vi "SDCP SMF Receiver and Trasmitter - Live Plot - Backup - v2.vi"() -> ()   [LabVIEW 2020]
uses:
  Typedefs/SDCP - Standard Message Frame Parameters - FGV - commands.ctl
  Typedefs/SDCP - Serial Port Control - Commands.ctl
panel:
  in  "Zero offset":bool
  out "Adjusted Offset":dbl
  in  "Offset":dbl(c297)
  out "Active Plot Names":string[](array[string])
  out "Value":dbl
  out "Time (ms)":dbl
  in  "Cursor Parameter":string(combo)
  out "Instantaeneous data":T1(array[cluster])
  in  "Time span (ms)":dbl
  in  "Channel 8 enable":bool
  in  "Channel 7 enable":bool
  in  "Channel 6 enable":bool
  in  "Channel 5 enable":bool
  in  "Channel 4 enable":bool
  in  "Channel 3 enable":bool
  in  "Channel 2 enable":bool
  in  "Channel 1 enable":bool
  in  "Channel 8 parameter":string(combo)
  in  "Channel 7 parameter":string(combo)
  in  "Channel 6 parameter":string(combo)
  in  "Channel 5 parameter":string(combo)
  in  "Channel 4 parameter":string(combo)
  in  "Channel 3 parameter":string(combo)
  in  "Channel 2 parameter":string(combo)
  in  "Channel 1 parameter":string(combo)
  in  "Plot file path":path
  out "Live Plot":T2(graph)
  out "Time (ms)":u32
  in  "Stop Application":bool
  in  "Trace file path":path
  in  "Baud rate":u32=9600
  in  "COM Port":refnum<visa-resource-name>
  in  "Parameter file path":path=path "E:/Projects/System Diagnostics and Control Protocol/SDCP_LabVIEW/Parameter Files/Motion_Processing.param"
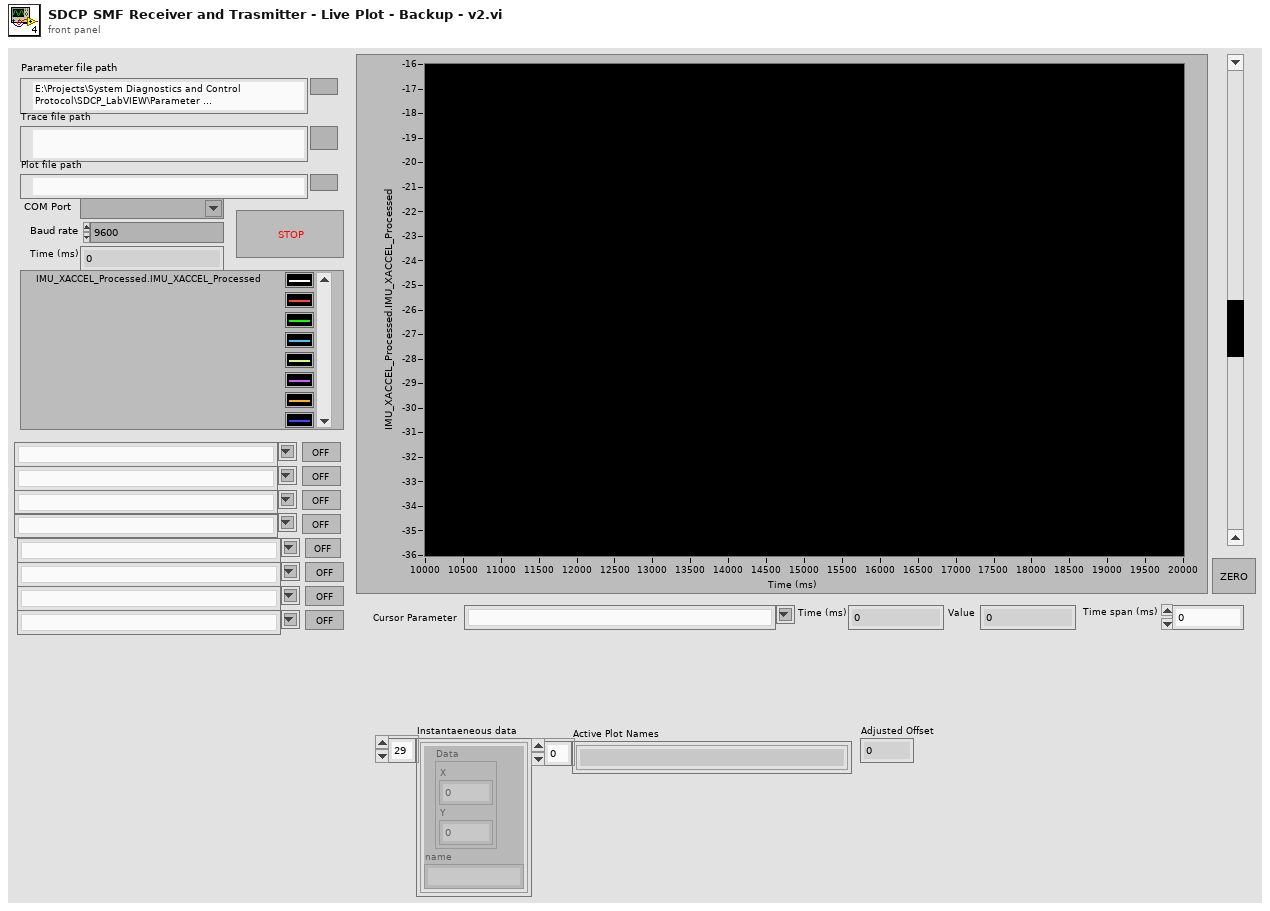
[diagram p1: front panel]
types:
  T1 = cluster{"Data":cluster{"X":dbl, "Y":dbl}, "name":string}[]
  T2 = cluster{"Plot data":cluster{"X":dbl, "Y":dbl}[]}[]
  T3 = typedef "SDCP - Serial Port Control - Commands.ctl" = enum16{"Open", "Read", "Write", "Get instance", "Close"}
  T4 = cluster{"data bytes":u8[], "Time (ms)":u32, "Direction":string}
  T5 = typedef "SDCP - Standard Message Frame Parameters - FGV - commands.ctl" = enum16{"Write descriptors", "Read descriptors", "Read values", "Load parameters from file", "Write values", "Read all descriptors"}
  T6 = typedef "SDCP - SMF parameter descriptors.ctl" = cluster{"Frame name":string, "Frame ID":i32, "Data type":string, "Start Position":i32, "Length":i32, "Factor":dbl, "Offset":dbl, "Parameter name":string, "Value":string}
  T7 = cluster{"name":string, "Data":cluster{"X":dbl, "Y":dbl}[]}
  T8 = cluster{"name":string, "Data":cluster{"X":dbl, "Y":dbl}[]}[]
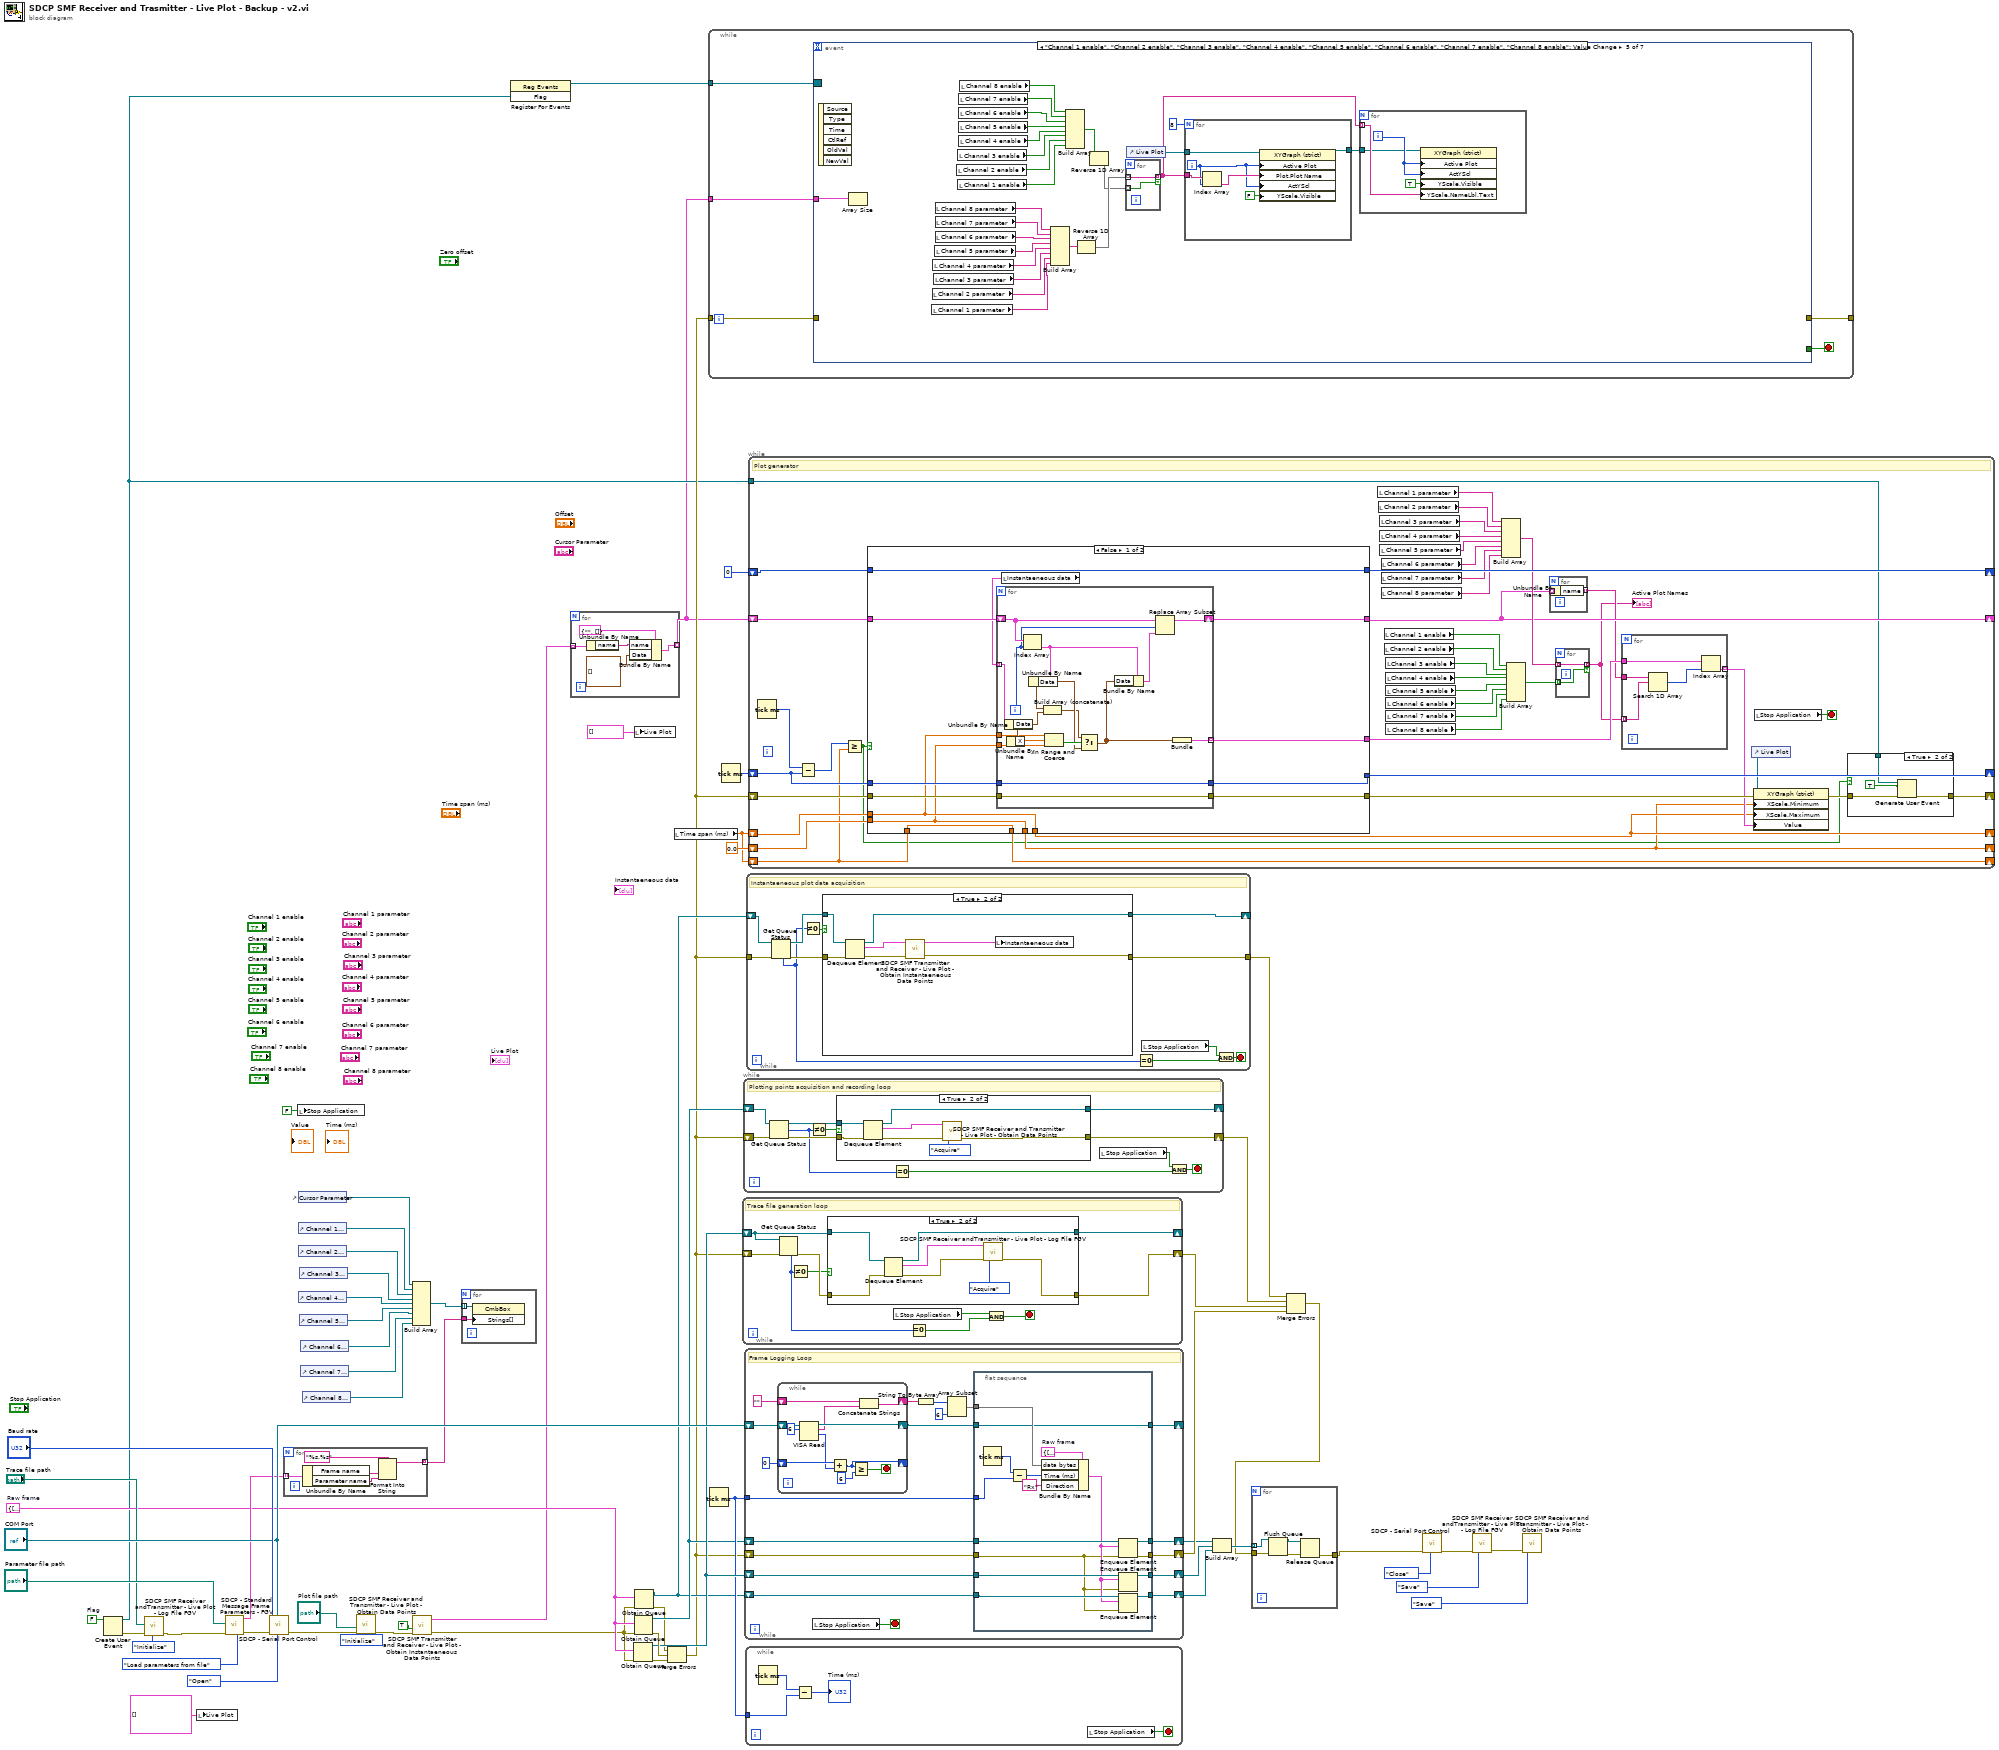
[diagram p0: block diagram]
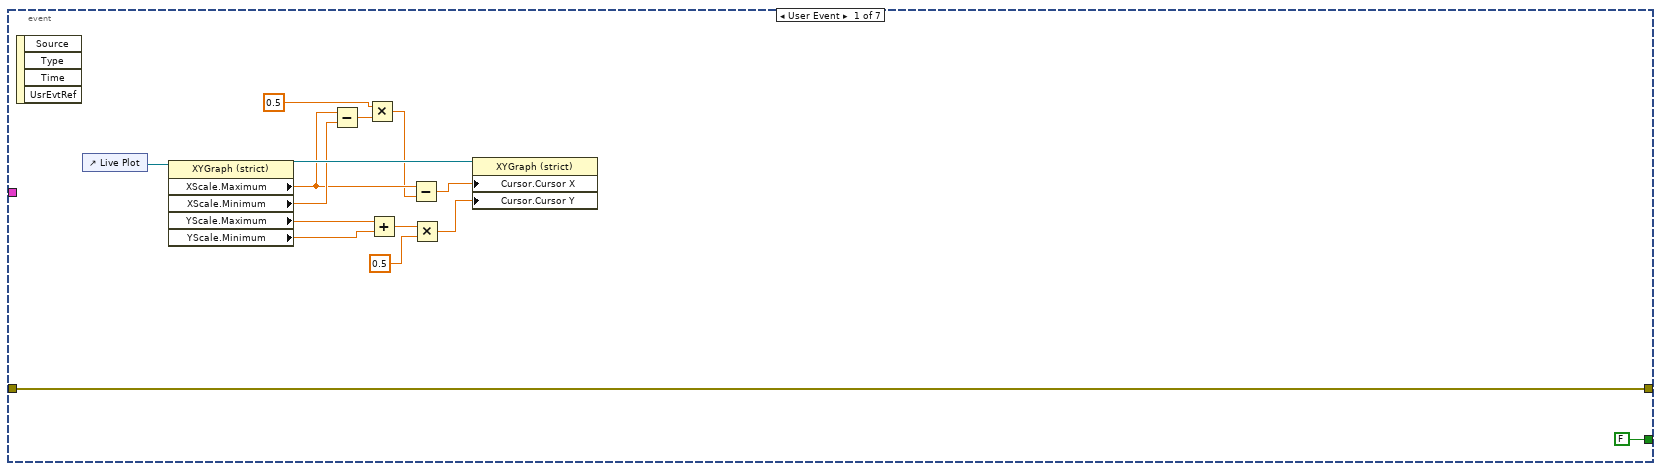
[diagram p2: hidden frame]
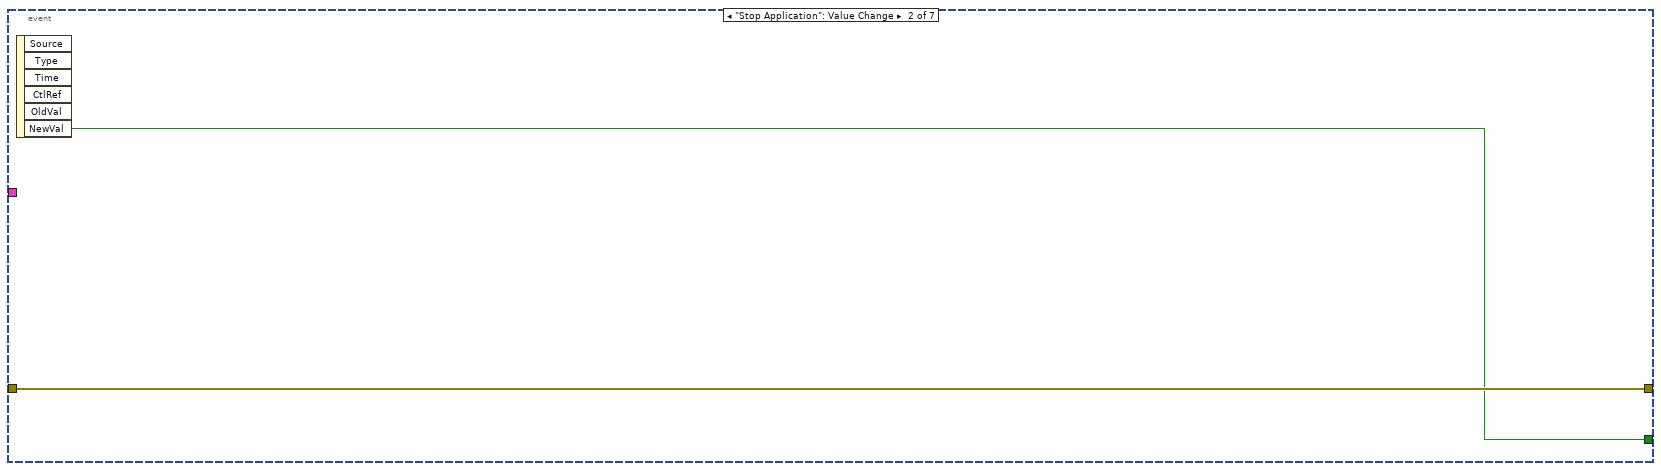
[diagram p3: hidden frame]
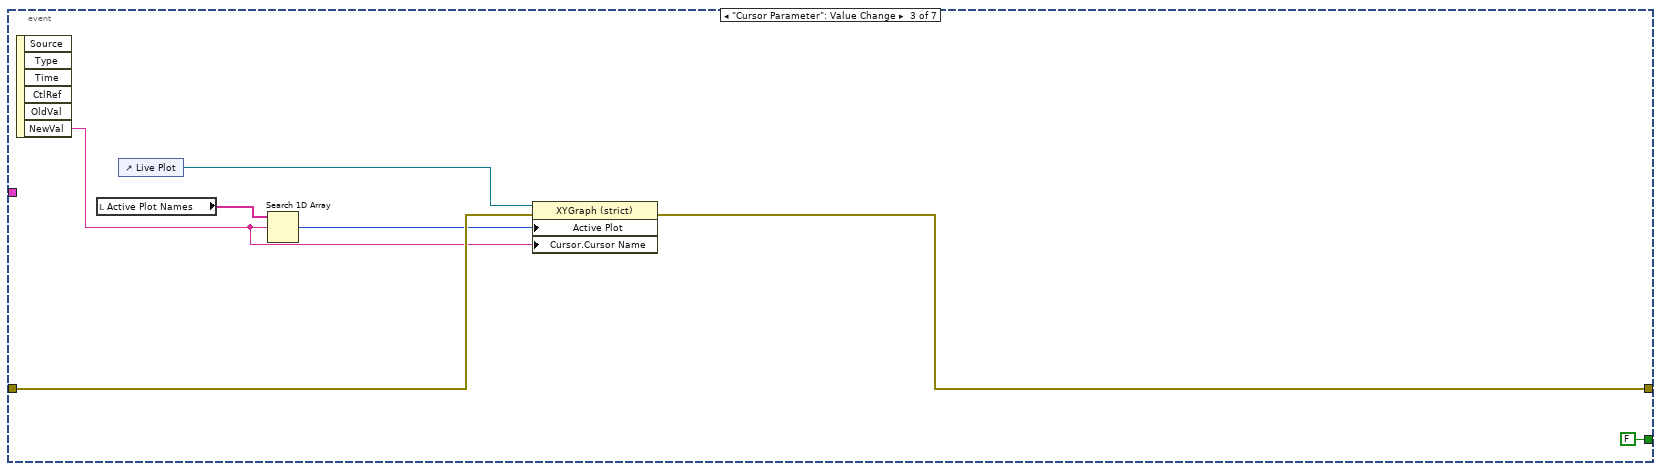
[diagram p4: hidden frame]
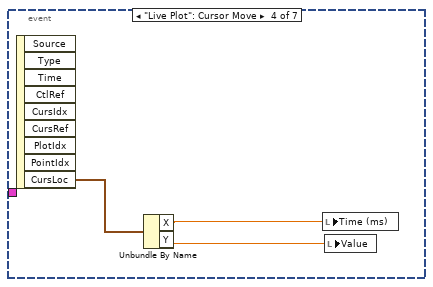
[diagram p5: hidden frame]
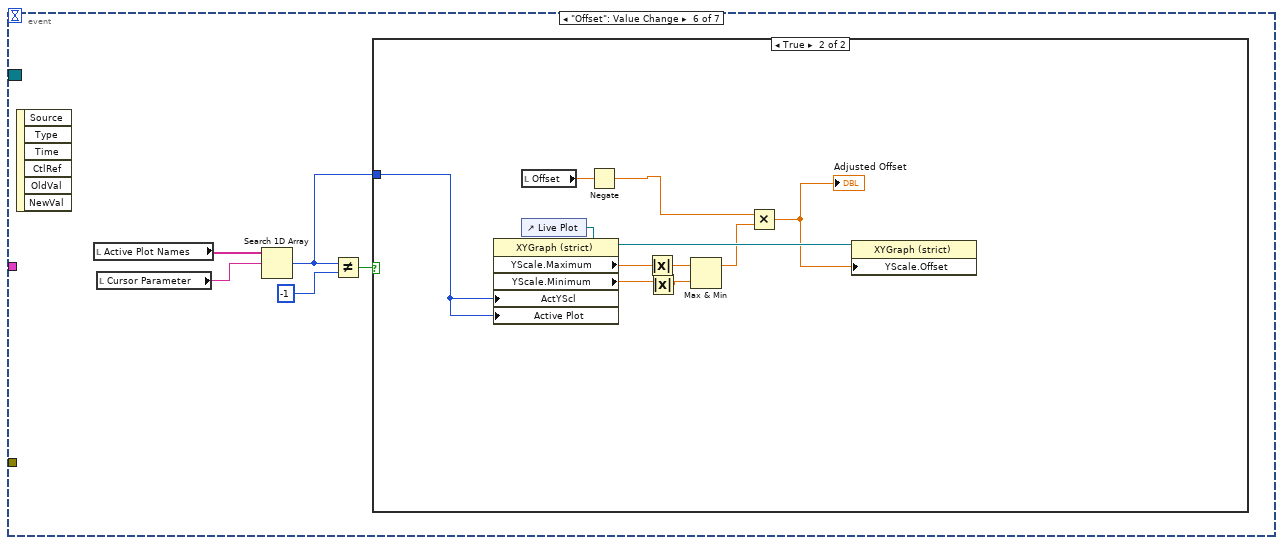
[diagram p6: hidden frame]
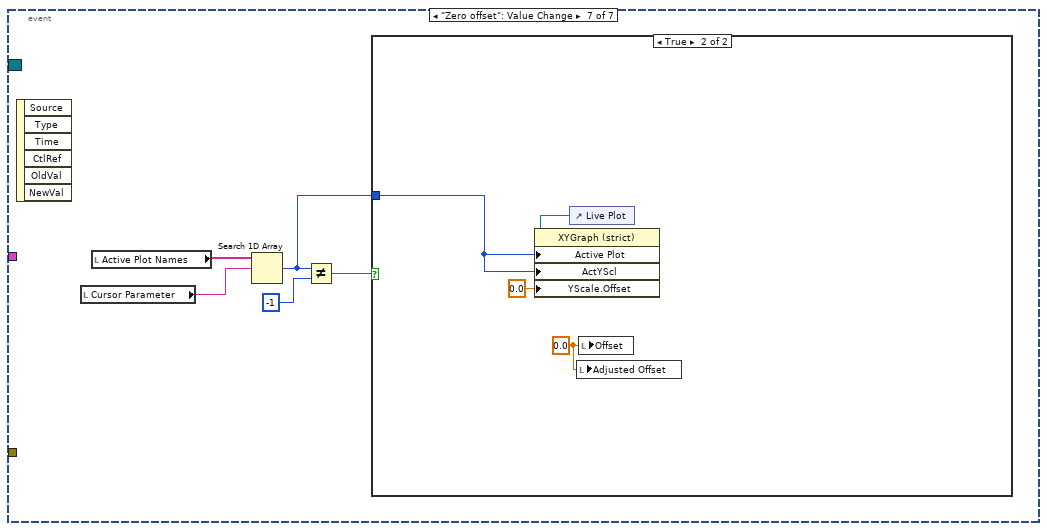
[diagram p8: hidden frame]
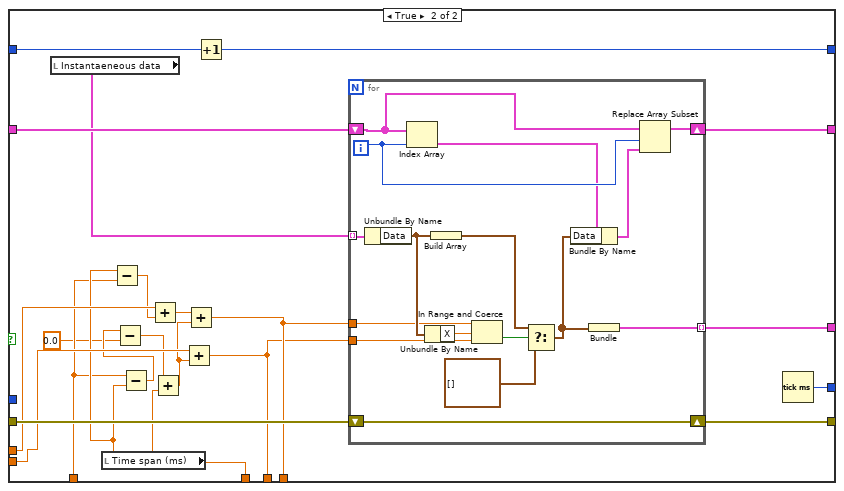
[diagram p11: hidden frame]
diagram:
  w4 = FALSE  # Flag
  w28 = T4 {"data bytes"=[], "Time (ms)"=0, "Direction"=""}  # Raw frame
  n1 = Create User Event(user event datatype=w4) -> (user event=w2:refnum<user-event>, error out=w5:errorcluster)  [unwired: 1 in]
  n2 = call "SDCP SMF Receiver andTransmitter - Live Plot - Log File FGV.vi"("error in (no error)"=w5, "Command"=enum16{"Initialize", "Acquire", "Save"}."Initialize", "Trace file path"="Trace file path") -> ("error out"=w46:errorcluster)  [unwired: 4 in]
  n3 = local write "Live Plot"(T2 [] ("Live Plot")) -> ()
  n4 = call "SDCP - Standard Message Frame Parameters - FGV.vi"("Parameter file path"="Parameter file path", "error in (no error)"=w46, "Command"=SDCP_-_Standard_Message_Frame_Parameters_-_FGV_-_commands."Load parameters from file") -> ("SMF Parameters descriptors out"=w41:T6[], "error out"=w62:errorcluster)  [unwired: 4 in]
  n5 = call "SDCP - Serial Port Control.vi"("Command"=SDCP_-_Serial_Port_Control_-_Commands."Open", "VISA resource name"="COM Port", "error in (no error)"=w62, "Baud rate"="Baud rate") -> ("error out"=w30:errorcluster)  [unwired: 4 in, 3 out]
  n6 = for {
    tunnel: w41 -> [w69] mode=indexing
    tunnel: [w65] -> w31 mode=indexing
    n7 = Unbundle By Name(w69) -> ("Frame name"=w67:string, "Parameter name"=w66:string)
    n8 = Format Into String(format string="%s.%s", w67, w66) -> (resulting string=w65:string)  [unwired: 2 in, 1 out]
  }
  n9 = local write "Stop Application"(FALSE ("Stop Application")) -> ()
  n10 = control-ref of="Cursor Parameter"() -> (w7:refnum<vi>)
  n11 = control-ref of="Channel 1 parameter"() -> (w40:refnum<vi>)
  n12 = control-ref of="Channel 2 parameter"() -> (w39:refnum<vi>)
  n13 = control-ref of="Channel 4 parameter"() -> (w37:refnum<vi>)
  n14 = control-ref of="Channel 3 parameter"() -> (w38:refnum<vi>)
  n15 = control-ref of="Channel 5 parameter"() -> (w36:refnum<vi>)
  n16 = control-ref of="Channel 6 parameter"() -> (w35:refnum<vi>)
  n17 = control-ref of="Channel 7 parameter"() -> (w34:refnum<vi>)
  n18 = control-ref of="Channel 8 parameter"() -> (w33:refnum<vi>)
  n19 = call "SDCP SMF Receiver and Transmitter - Live Plot - Obtain Data Points.vi"("error in (no error)"=w30, "Plot file path"="Plot file path", "Command"=enum16{"Initialize", "Acquire", "Save"}."Initialize") -> ("error out"=w17:errorcluster)  [unwired: 4 in]
  n20 = Build Array(w7, w40, w39, w38, w37, w36, w35, w34, w33) -> (w32:refnum<vi>[])
  n21 = call "SDCP SMF Transmitter and Receiver - Live Plot - Obtain Instantaeneous Data Points.vi"("Initialize ?"=TRUE, "error in (no error)"=w17) -> ("Instantaeneous data"=w13:T1, "error out"=w16:errorcluster)  [unwired: 4 in]
  n22 = for {
    tunnel: w32 -> [w71] mode=indexing
    tunnel: w31 -> [w70]
    n23 = property class="CmbBox"(reference=w71, "Strings[]"=w70) -> ()  [unwired: 1 in, 2 out]
  }
  n24 = register-events(w2) -> (reference out=w3:refnum<event-registration>)  [unwired: 2 in, 1 out]
  n25 = for {
    tunnel: w13 -> [w76] mode=indexing
    tunnel: [w73] -> w1 mode=indexing
    n26 = Unbundle By Name(w76) -> ("name"=w74:string)
    n27 = Bundle By Name(cluster=T7 {"name"="", "Data"=[]}, "name"=w74, "Data"=cluster{"X":dbl, "Y":dbl}[] []) -> (w73:T7)
  }
  n28 = Obtain Queue(element data type=w28, error in (no error)=w16) -> (queue out=w56:refnum<queue>, error out=w57:errorcluster)  [unwired: 3 in, 1 out]
  n29 = local write "Live Plot"(cluster{"Data":cluster{"X":dbl, "Y":dbl}[]}[] []) -> ()
  n30 = Obtain Queue(element data type=w28, error in (no error)=w16) -> (queue out=w47:refnum<queue>, error out=w58:errorcluster)  [unwired: 3 in, 1 out]
  n31 = Obtain Queue(element data type=w28, error in (no error)=w16) -> (queue out=w19:refnum<queue>, error out=w27:errorcluster)  [unwired: 3 in, 1 out]
  n32 = Merge Errors(w27, w58, w57) -> (w6:errorcluster)
  n33 = local read "Time span (ms)"() -> (w8:dbl)
  n34 = while {
    tunnel: w6 -> [w81]
    tunnel: [w80] -> _
    tunnel: w3 -> [w78]
    tunnel: w1 -> [w77]
    stop <- w79 stop-if-true
    n35 = event shown="[4] \"Channel 1 enable\", \"Channel 2 enable\", \"Channel 3 enable\", \"Channel 4 enable\", \"Channel 5 enable\", \"Channel 6 enable\", \"Channel 7 enable\", \"Channel 8 enable\": Value Change" {
      selector: w78 -> [_ _ _ _ _ _ _]
      dyn-events: _ -> [_ _ _ _ _ _ _]
      timeout: _ -> [_ _ _ _ _ _ _]
      tunnel: w81 -> [w96 w98 w104 _ _ _ _]
      tunnel: [w96 w98 w100 _ _ _ _] -> w80
      tunnel: [FALSE w97 FALSE ("NewVal") _ _ _ _] -> w79
      tunnel: w77 -> [_ _ _ _ w117 _ _]
      event User Event {
        n36 = event-data() -> ()  [unwired: 1 in, 4 out]
        n37 = control-ref of="Live Plot"() -> (w94:refnum<vi>)
        n38 = property class="XYGraph (strict)"(reference=w94) -> (reference out=w89:refnum<vi>, "XScale.Maximum"=w86:dbl, "XScale.Minimum"=w87:dbl, "YScale.Maximum"=w93:dbl, "YScale.Minimum"=w92:dbl)  [unwired: 1 in, 1 out]
        n39 = Subtract(x=w86, y=w87) -> (x-y=w85:dbl)
        n40 = Multiply(x=0.5, y=w85) -> (x*y=w83:dbl)
        n41 = Add(x=w93, y=w92) -> (x+y=w91:dbl)
        n42 = Subtract(x=w86, y=w83) -> (x-y=w82:dbl)
        n43 = Multiply(x=w91, y=0.5) -> (x*y=w88:dbl)
        n44 = property class="XYGraph (strict)"(reference=w89, "Cursor.Cursor X"=w82, "Cursor.Cursor Y"=w88) -> ()  [unwired: 1 in, 2 out]
      }
      event "Stop Application": Value Change {
        n45 = event-data() -> ("NewVal"=w97:bool)  [unwired: 1 in, 5 out]
      }
      event "Cursor Parameter": Value Change {
        n46 = event-data() -> ("NewVal"=w101:string)  [unwired: 1 in, 5 out]
        n47 = local read "Active Plot Names"() -> (w99:string[])
        n48 = control-ref of="Live Plot"() -> (w103:refnum<vi>)
        n49 = Search 1D Array(1D array=w99, element=w101) -> (index of element=w102:i32)  [unwired: 1 in]
        n50 = property class="XYGraph (strict)"(reference=w103, error in=w104, "Active Plot"=w102, "Cursor.Cursor Name"=w101) -> (error out=w100:errorcluster)  [unwired: 1 out]
      }
      event "Live Plot": Cursor Move {
        n51 = event-data() -> ("CursLoc"=w108:cluster{"X":dbl, "Y":dbl})  [unwired: 1 in, 8 out]
        n52 = Unbundle By Name(w108) -> ("X"=w107:dbl, "Y"=w106:dbl)
        n53 = local write "Time (ms)"(w107) -> ()
        n54 = local write "Value"(w106) -> ()
      }
      event "Channel 1 enable", "Channel 2 enable", "Channel 3 enable", "Channel 4 enable", "Channel 5 enable", "Channel 6 enable", "Channel 7 enable", "Channel 8 enable": Value Change {
        n55 = event-data() -> ()  [unwired: 1 in, 6 out]
        n56 = Array Size(array=w117) -> ()  [unwired: 1 out]
        n57 = local read "Channel 1 parameter"() -> (w118:string)
        n58 = local read "Channel 2 parameter"() -> (w119:string)
        n59 = local read "Channel 4 parameter"() -> (w121:string)
        n60 = local read "Channel 3 parameter"() -> (w120:string)
        n61 = local read "Channel 5 parameter"() -> (w122:string)
        n62 = local read "Channel 8 parameter"() -> (w125:string)
        n63 = local read "Channel 7 parameter"() -> (w124:string)
        n64 = local read "Channel 6 parameter"() -> (w123:string)
        n65 = local read "Channel 2 enable"() -> (w127:bool)
        n66 = local read "Channel 3 enable"() -> (w128:bool)
        n67 = local read "Channel 1 enable"() -> (w126:bool)
        n68 = local read "Channel 7 enable"() -> (w132:bool)
        n69 = local read "Channel 6 enable"() -> (w131:bool)
        n70 = local read "Channel 5 enable"() -> (w130:bool)
        n71 = local read "Channel 4 enable"() -> (w129:bool)
        n72 = local read "Channel 8 enable"() -> (w133:bool)
        n73 = Build Array(w125, w124, w123, w122, w121, w120, w119, w118) -> (w115:string[])
        n74 = Build Array(w133, w132, w131, w130, w129, w128, w127, w126) -> (w114:bool[])
        n75 = Reverse 1D Array(array=w115) -> (reversed array=w112:string[])
        n76 = Reverse 1D Array(array=w114) -> (reversed array=w111:bool[])
        n77 = for {
          tunnel: w112 -> [w145] mode=indexing
          tunnel: w111 -> [w144] mode=indexing
          tunnel: [w145] -> w110 mode=indexing if=w144
        }
        n78 = control-ref of="Live Plot"() -> (w113:refnum<vi>)
        n79 = for {
          N: 8 -> [_]
          tunnel: w113 -> [w143]
          tunnel: w110 -> [w142]
          tunnel: [w140] -> w109
          i -> [w139]
          n80 = Index Array(array=w142, index=w139) -> (element=w141:string)
          n81 = property class="XYGraph (strict)"(reference=w143, "Active Plot"=w139, "Plot.Plot Name"=w141, "ActYScl"=w139, "YScale.Visible"=FALSE ("Y Scale.Visible")) -> (reference out=w140:refnum<vi>)  [unwired: 1 in, 1 out]
        }
        n82 = for {
          tunnel: w110 -> [w136] mode=indexing
          tunnel: w109 -> [w134]
          i -> [w137]
          n83 = property class="XYGraph (strict)"(reference=w134, "Active Plot"=w137, "ActYScl"=w137, "YScale.Visible"=TRUE ("Y Scale.Visible"), "YScale.NameLbl.Text"=w136) -> ()  [unwired: 1 in, 2 out]
        }
      }
      event "Offset": Value Change {
        n84 = event-data() -> ()  [unwired: 1 in, 6 out]
        n85 = local read "Active Plot Names"() -> (w150:string[])
        n86 = local read "Cursor Parameter"() -> (w149:string)
        n87 = Search 1D Array(1D array=w150, element=w149) -> (index of element=w146:i32)  [unwired: 1 in]
        n88 = Not Equal?(x=w146, y=-1) -> (x != y?=w147:bool)
        n89 = case shown="True" w147 {
          tunnel: w146 -> [_ w160]
          frame False {
          }
          frame True {
            n90 = local read "Offset"() -> (w159:dbl)
            n91 = control-ref of="Live Plot"() -> (w161:refnum<vi>)
            n92 = property class="XYGraph (strict)"(reference=w161, "ActYScl"=w160, "Active Plot"=w160) -> (reference out=w154:refnum<vi>, "YScale.Maximum"=w158:dbl, "YScale.Minimum"=w157:dbl)  [unwired: 1 in, 1 out]
            n93 = Negate(x=w159) -> (-x=w153:dbl)
            n94 = Absolute Value(x=w158) -> (abs(x)=w156:dbl)
            n95 = Absolute Value(x=w157) -> (abs(x)=w155:dbl)
            n96 = Max & Min(x=w156, y=w155) -> (max(x,y)=w152:dbl)  [unwired: 1 out]
            n97 = Multiply(x=w153, y=w152) -> (x*y=w151:dbl)
            "Adjusted Offset" <- w151
            n98 = property class="XYGraph (strict)"(reference=w154, "YScale.Offset"=w151) -> ()  [unwired: 1 in, 2 out]
          }
        }
      }
      event "Zero offset": Value Change {
        n99 = event-data() -> ()  [unwired: 1 in, 6 out]
        n100 = local read "Cursor Parameter"() -> (w165:string)
        n101 = local read "Active Plot Names"() -> (w166:string[])
        n102 = Search 1D Array(1D array=w166, element=w165) -> (index of element=w162:i32)  [unwired: 1 in]
        n103 = Not Equal?(x=w162, y=-1) -> (x != y?=w163:bool)
        n104 = case shown="True" w163 {
          tunnel: w162 -> [_ w169]
          frame False {
          }
          frame True {
            w167 = 0.0 ("Offset")
            n105 = control-ref of="Live Plot"() -> (w170:refnum<vi>)
            n106 = property class="XYGraph (strict)"(reference=w170, "Active Plot"=w169, "ActYScl"=w169, "YScale.Offset"=0.0 ("Y Scale.Offset and Multiplier:Offset")) -> ()  [unwired: 1 in, 2 out]
            n107 = local write "Adjusted Offset"(w167) -> ()
            n108 = local write "Offset"(w167) -> ()
          }
        }
      }
    }
  }
  n109 = Tick Count (ms)() -> (millisecond timer value=w48:u32)
  n110 = Tick Count (ms)() -> (millisecond timer value=w14:u32)
  n111 = while {
    shift-right: [w178] -> w50
    shift-left: w6 -> [w180]
    shift-right: [w177] -> _
    shift-left: w56 -> [w179]
    stop <- w173 stop-if-true
    # "Trace file generation loop"
    n112 = Get Queue Status(queue=w179, error in (no error)=w180) -> (error out=w176:errorcluster, # elements in queue=w172:i32)  [unwired: 1 in, 6 out]
    n113 = Not Equal To 0?(x=w172) -> (x != 0?=w175:bool)
    n114 = case shown="True" w175 {
      tunnel: w176 -> [w182 w187]
      tunnel: [w182 w189] -> w178
      tunnel: w179 -> [w181 w185]
      tunnel: [w181 w184] -> w177
      frame False {
      }
      frame True {
        n115 = Dequeue Element(queue=w185, error in (no error)=w187) -> (queue out=w184:refnum<queue>, element=w183:T4, error out=w186:errorcluster)  [unwired: 1 in, 1 out]
        n116 = call "SDCP SMF Receiver andTransmitter - Live Plot - Log File FGV.vi"("error in (no error)"=w186, "Command"=enum16{"Initialize", "Acquire", "Save"}."Acquire", "Raw frame"=w183) -> ("error out"=w189:errorcluster)  [unwired: 4 in]
      }
    }
    n117 = local read "Stop Application"() -> (w174:bool)
    n118 = Equal To 0?(x=w172) -> (x = 0?=w171:bool)
    n119 = And(x=w174, y=w171) -> (x .and. y?=w173:bool)
  }
  n120 = while {
    shift-right: [w194] -> _
    shift-left: w47 -> [w199]
    shift-right: [w196] -> w26
    shift-left: w6 -> [w200]
    stop <- w192 stop-if-true
    # "Plotting points acquisition and recording loop"
    n121 = Get Queue Status(queue=w199, error in (no error)=w200) -> (queue out=w195:refnum<queue>, error out=w197:errorcluster, # elements in queue=w193:i32)  [unwired: 1 in, 5 out]
    n122 = Not Equal To 0?(x=w193) -> (x != 0?=w198:bool)
    n123 = case shown="True" w198 {
      tunnel: w197 -> [w202 w209]
      tunnel: [w202 w204] -> w196
      tunnel: w195 -> [w201 w208]
      tunnel: [w201 w207] -> w194
      frame False {
      }
      frame True {
        n124 = Dequeue Element(queue=w208, error in (no error)=w209) -> (queue out=w207:refnum<queue>, element=w205:T4, error out=w206:errorcluster)  [unwired: 1 in, 1 out]
        n125 = call "SDCP SMF Receiver and Transmitter - Live Plot - Obtain Data Points.vi"("error in (no error)"=w206, "Command"=enum16{"Initialize", "Acquire", "Save"}."Acquire", "Raw frame"=w205) -> ("error out"=w204:errorcluster)  [unwired: 4 in]
      }
    }
    n126 = Equal To 0?(x=w193) -> (x = 0?=w190:bool)
    n127 = local read "Stop Application"() -> (w191:bool)
    n128 = And(x=w191, y=w190) -> (x .and. y?=w192:bool)
  }
  n129 = while {
    tunnel: w48 -> [w221]
    shift-right: [w217] -> _
    shift-left: "COM Port" -> [w228]
    shift-right: [w219] -> w49
    shift-left: w6 -> [w220]
    shift-right: [w215] -> w25
    shift-left: w47 -> [w216]
    shift-right: [w213] -> w24
    shift-left: w56 -> [w214]
    shift-right: [w210] -> w23
    shift-left: w19 -> [w211]
    stop <- w212 stop-if-true
    # "Frame Logging Loop"
    n130 = while {
      shift-right: [w254] -> w218
      shift-left: w228 -> [w255]
      shift-right: [w246] -> w225
      shift-left: "" -> [w248]
      shift-right: [w250] -> _
      shift-left: 0 -> [w253]
      stop <- w249 stop-if-true
      n131 = VISA Read(VISA resource name=w255, byte count=u32 6) -> (VISA resource name out=w254:refnum<visa-resource-name>, read buffer=w247:string, return count=w252:u32)  [unwired: 1 in, 1 out]
      n132 = Add(x=w253, y=w252) -> (x+y=w250:u32)
      n133 = Greater Or Equal?(x=w250, y=u32 6) -> (x >= y?=w249:bool)
      n134 = Concatenate Strings(w248, w247) -> (w246:string)
    }
    n135 = local read "Stop Application"() -> (w212:bool)
    n136 = String To Byte Array(string=w225) -> (unsigned byte array=w224:u8[])
    n137 = Array Subset(array=w224, length=6) -> (w222:u8[])  [unwired: 1 in]
    n138 = flat-sequence {
      tunnel: w222 -> [w234]
      tunnel: w221 -> [w243]
      tunnel: w220 -> [w229]
      tunnel: [w240] -> w219
      tunnel: w218 -> [w233]
      tunnel: [w233] -> w217
      tunnel: w216 -> [w239]
      tunnel: [w238] -> w215
      tunnel: w214 -> [w237]
      tunnel: [w236] -> w213
      tunnel: w211 -> [w232]
      tunnel: [w230] -> w210
      frame #0 {
        w242 = T4 {"data bytes"=[], "Time (ms)"=0, "Direction"=""}  # Raw frame
        n139 = Tick Count (ms)() -> (millisecond timer value=w244:u32)
        n140 = Subtract(x=w244, y=w243) -> (x-y=w241:u32)
        n141 = Bundle By Name(cluster=w242, "data bytes"=w234, "Time (ms)"=w241, "Direction"="Rx") -> (w231:T4)
        n142 = Enqueue Element(queue=w239, element=w231, error in (no error)=w229) -> (queue out=w238:refnum<queue>, error out=w240:errorcluster)  [unwired: 1 in, 1 out]
        n143 = Enqueue Element(queue=w237, element=w231, error in (no error)=w229) -> (queue out=w236:refnum<queue>)  [unwired: 1 in, 2 out]
        n144 = Enqueue Element(queue=w232, element=w231, error in (no error)=w229) -> (queue out=w230:refnum<queue>)  [unwired: 1 in, 2 out]
      }
    }
  }
  n145 = while {
    tunnel: w48 -> [w258]
    stop <- w256 stop-if-true
    n146 = Tick Count (ms)() -> (millisecond timer value=w259:u32)
    n147 = Subtract(x=w259, y=w258) -> (x-y=→"Time (ms)":u32)
    n148 = local read "Stop Application"() -> (w256:bool)
  }
  n149 = while {
    shift-right: [w262] -> _
    shift-left: w19 -> [w269]
    tunnel: w6 -> [w270]
    tunnel: [w261] -> w18
    stop <- w265 stop-if-true
    # "Instantaeneous plot data acquisition"
    n150 = Get Queue Status(queue=w269, error in (no error)=w270) -> (queue out=w263:refnum<queue>, error out=w264:errorcluster, # elements in queue=w260:i32)  [unwired: 1 in, 5 out]
    n151 = Not Equal To 0?(x=w260) -> (x != 0?=w268:bool)
    n152 = case shown="True" w268 {
      tunnel: w264 -> [w271 w279]
      tunnel: w263 -> [w272 w278]
      tunnel: [w272 w277] -> w262
      tunnel: [w271 w274] -> w261
      frame False {
      }
      frame True {
        n153 = Dequeue Element(queue=w278, error in (no error)=w279) -> (queue out=w277:refnum<queue>, element=w275:T4, error out=w276:errorcluster)  [unwired: 1 in, 1 out]
        n154 = call "SDCP SMF Transmitter and Receiver - Live Plot - Obtain Instantaeneous Data Points.vi"("Raw frame"=w275, "error in (no error)"=w276) -> ("Instantaeneous data"=w273:T1, "error out"=w274:errorcluster)  [unwired: 4 in]
        n155 = local write "Instantaeneous data"(w273) -> ()
      }
    }
    n156 = Equal To 0?(x=w260) -> (x = 0?=w267:bool)
    n157 = local read "Stop Application"() -> (w266:bool)
    n158 = And(x=w266, y=w267) -> (x .and. y?=w265:bool)
  }
  n159 = while {
    shift-right: [w283] -> _
    shift-left: w6 -> [w320]
    shift-right: [w319] -> _
    shift-left: w14 -> [w317]
    shift-right: [w292] -> _
    shift-left: w1 -> [w318]
    shift-right: [w316] -> _
    shift-left: 0 -> [w315]
    shift-right: [w290] -> _
    shift-left: w8 -> [w289]
    shift-right: [w287] -> _
    shift-left: 0.0 -> [w288]
    shift-right: [w286] -> _
    shift-left: w8 -> [w285]
    tunnel: w2 -> [w282]
    stop <- w323 stop-if-true
    # "Plot generator"
    n160 = Tick Count (ms)() -> (millisecond timer value=w322:u32)
    n161 = Subtract(x=w322, y=w317) -> (x-y=w321:u32)
    n162 = Greater Or Equal?(x=w321, y=w285) -> (x >= y?=w281:bool)
    n163 = case shown="False" w281 {
      tunnel: w320 -> [w344 w382]
      tunnel: [w343 w383] -> w314
      tunnel: [w346 w387] -> w319
      tunnel: w318 -> [w349 w386]
      tunnel: [w345 w384] -> w292
      tunnel: w317 -> [w347 _]
      tunnel: [w341 w381] -> w294
      tunnel: w315 -> [w342 w380]
      tunnel: [w342 w379] -> w316
      tunnel: [w340 w376] -> w290
      tunnel: [w339 w375] -> w287
      tunnel: w289 -> [w340 w378]
      tunnel: w288 -> [w339 w377]
      tunnel: [w338 w373] -> w286
      tunnel: w285 -> [w338 w372]
      frame False {
        n164 = local read "Instantaeneous data"() -> (w348:T1)
        n165 = for {
          shift-right: [w361] -> w345
          shift-left: w349 -> [w364]
          tunnel: w348 -> [w365] mode=indexing
          tunnel: w347 -> [w360]
          tunnel: [w360] -> w346
          tunnel: w344 -> [w359]
          tunnel: [w359] -> w343
          tunnel: [w358] -> w341 mode=indexing
          tunnel: w340 -> [w351]
          tunnel: w339 -> [w350]
          i -> [w363]
          n166 = Unbundle By Name(w365) -> ("Data"=w354:cluster{"X":dbl, "Y":dbl})
          n167 = Unbundle By Name(w354) -> ("X"=w357:dbl)
          n168 = Index Array(array=w364, index=w363) -> (element=w366:T7)
          n169 = Unbundle By Name(w366) -> ("Data"=w355:cluster{"X":dbl, "Y":dbl}[])
          n170 = Build Array (concatenate)(w355, w354) -> (w353:cluster{"X":dbl, "Y":dbl}[])
          n171 = In Range and Coerce(upper limit=w351, x=w357, lower limit=w350) -> (In Range?=w356:bool)  [unwired: 1 out]
          n172 = Select(t=w353, s=w356, f=w355) -> (s? t:f=w352:cluster{"X":dbl, "Y":dbl}[])
          n173 = Bundle By Name(cluster=w366, "Data"=w352) -> (w362:T7)
          n174 = Replace Array Subset(array=w364, new element=w362, index=w363) -> (w361:T8)
          n175 = Bundle("Data"=w352) -> (w358:cluster{"Data":cluster{"X":dbl, "Y":dbl}[]})  [unwired: 1 in]
        }
      }
      frame True {
        n176 = local read "Instantaeneous data"() -> (w385:T1)
        n177 = local read "Time span (ms)"() -> (w373:dbl)
        n178 = Subtract(x=w373, y=w372) -> (x-y=w370:dbl)
        n179 = Subtract(x=w372, y=w373) -> (x-y=w369:dbl)
        n180 = Subtract(x=w369, y=0.0) -> (x-y=w368:dbl)
        n181 = Add(x=w378, y=w370) -> (x+y=w371:dbl)
        n182 = Add(x=w368, y=w373) -> (x+y=w374:dbl)
        n183 = Add(x=w377, y=w374) -> (x+y=w375:dbl)
        n184 = Add(x=w371, y=w374) -> (x+y=w376:dbl)
        n185 = Increment(x=w380) -> (x+1=w379:i32)
        n186 = for {
          shift-right: [w394] -> w384
          shift-left: w386 -> [w403]
          tunnel: w385 -> [w401] mode=indexing
          shift-right: [w398] -> w383
          shift-left: w382 -> [w398]
          tunnel: [w397] -> w381 mode=indexing
          tunnel: w376 -> [w389]
          tunnel: w375 -> [w388]
          i -> [w402]
          n187 = Unbundle By Name(w401) -> ("Data"=w396:cluster{"X":dbl, "Y":dbl})
          n188 = Index Array(array=w403, index=w402) -> (element=w400:T7)
          n189 = Unbundle By Name(w396) -> ("X"=w395:dbl)
          n190 = Build Array(w396) -> (w392:cluster{"X":dbl, "Y":dbl}[])
          n191 = In Range and Coerce(upper limit=w389, x=w395, lower limit=w388) -> (In Range?=w393:bool)  [unwired: 1 out]
          n192 = Select(t=w392, s=w393, f=cluster{"X":dbl, "Y":dbl}[] []) -> (s? t:f=w391:cluster{"X":dbl, "Y":dbl}[])
          n193 = Bundle By Name(cluster=w400, "Data"=w391) -> (w399:T7)
          n194 = Bundle("f"=w391) -> (w397:cluster{"f":cluster{"X":dbl, "Y":dbl}[]})  [unwired: 1 in]
          n195 = Replace Array Subset(array=w403, new element=w399, index=w402) -> (w394:T8)
        }
        n196 = Tick Count (ms)() -> (millisecond timer value=w387:u32)
      }
    }
    n197 = local read "Channel 1 parameter"() -> (w312:string)
    n198 = local read "Channel 2 parameter"() -> (w311:string)
    n199 = local read "Channel 3 parameter"() -> (w310:string)
    n200 = local read "Channel 4 parameter"() -> (w309:string)
    n201 = local read "Channel 5 parameter"() -> (w308:string)
    n202 = local read "Channel 6 parameter"() -> (w307:string)
    n203 = local read "Channel 7 parameter"() -> (w306:string)
    n204 = local read "Channel 8 parameter"() -> (w305:string)
    n205 = local read "Channel 1 enable"() -> (w304:bool)
    n206 = local read "Channel 2 enable"() -> (w303:bool)
    n207 = local read "Channel 3 enable"() -> (w302:bool)
    n208 = local read "Channel 4 enable"() -> (w301:bool)
    n209 = local read "Channel 5 enable"() -> (w300:bool)
    n210 = local read "Channel 6 enable"() -> (w299:bool)
    n211 = local read "Channel 7 enable"() -> (w298:bool)
    n212 = local read "Channel 8 enable"() -> (w297:bool)
    n213 = Build Array(w312, w311, w310, w309, w308, w307, w306, w305) -> (w295:string[])
    n214 = Build Array(w304, w303, w302, w301, w300, w299, w298, w297) -> (w296:bool[])
    n215 = for {
      tunnel: w292 -> [w330] mode=indexing
      tunnel: [w329] -> w291 mode=indexing
      n216 = Unbundle By Name(w330) -> ("name"=w329:string)
    }
    n217 = for {
      tunnel: w296 -> [w336] mode=indexing
      tunnel: w295 -> [w337] mode=indexing
      tunnel: [w337] -> w280 mode=indexing if=w336
    }
    "Active Plot Names" <- w280
    n218 = for {
      tunnel: w280 -> [w332] mode=indexing
      tunnel: w294 -> [w335]
      tunnel: [w333] -> w293 mode=indexing
      tunnel: w291 -> [w331]
      n219 = Search 1D Array(1D array=w331, element=w332) -> (index of element=w334:i32)  [unwired: 1 in]
      n220 = Index Array(array=w335, index=w334) -> (element=w333:cluster{"f":cluster{"X":dbl, "Y":dbl}[]})
    }
    n221 = control-ref of="Live Plot"() -> (w313:refnum<vi>)
    n222 = property class="XYGraph (strict)"(reference=w313, error in=w314, "XScale.Minimum"=w287, "XScale.Maximum"=w290, "Value"=w293) -> (error out=w284:errorcluster)  [unwired: 1 out]
    n223 = local read "Stop Application"() -> (w323:bool)
    n224 = case shown="True" w281 {
      tunnel: w284 -> [w324 w328]
      tunnel: [w324 w327] -> w283
      tunnel: w282 -> [_ w325]
      frame False {
      }
      frame True {
        n225 = Generate User Event(user event=w325, event data cluster=TRUE, error in=w328) -> (error out=w327:errorcluster)  [unwired: 1 in, 1 out]
      }
    }
  }
  n226 = Build Array(w25, w24, w23) -> (w22:refnum<queue>[])
  n227 = Merge Errors(w18, w26, w50, w49) -> (w21:errorcluster)
  n228 = for {
    tunnel: w22 -> [w407] mode=indexing
    tunnel: w21 -> [w408]
    tunnel: [w404] -> w20
    n229 = Flush Queue(queue=w407, error in (no error)=w408) -> (queue out=w405:refnum<queue>, error out=w406:errorcluster)  [unwired: 1 out]
    n230 = Release Queue(queue=w405, error in (no error)=w406) -> (error out=w404:errorcluster)  [unwired: 1 in, 2 out]
  }
  n231 = call "SDCP - Serial Port Control.vi"("Command"=SDCP_-_Serial_Port_Control_-_Commands."Close", "error in (no error)"=w20) -> ("error out"=w52:errorcluster)  [unwired: 6 in, 3 out]
  n232 = call "SDCP SMF Receiver andTransmitter - Live Plot - Log File FGV.vi"("error in (no error)"=w52, "Command"=enum16{"Initialize", "Acquire", "Save"}."Save") -> ("error out"=w43:errorcluster)  [unwired: 5 in]
  n233 = call "SDCP SMF Receiver and Transmitter - Live Plot - Obtain Data Points.vi"("error in (no error)"=w43, "Command"=enum16{"Initialize", "Acquire", "Save"}."Save") -> ()  [unwired: 5 in, 1 out]
